vi "ShiftWristSetpoints.vi"(1 "Grab Hatch":bool, 2 "Setpoints":dbl[](array[numeric])) -> (0 "Setpoints Out":dbl[](array[numeric]))   [LabVIEW 2018]
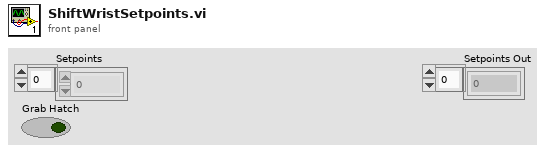
[diagram p1: front panel]
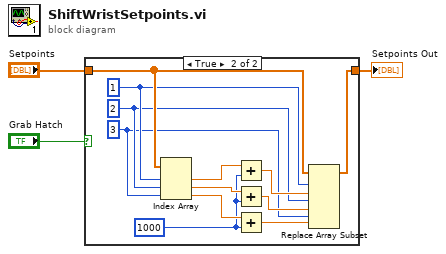
[diagram p0: block diagram]
diagram:
  n1 = case shown="True" "Grab Hatch" {
    tunnel: "Setpoints" -> [w4 w16]
    tunnel: [w4 w5] -> w2
    frame False {
    }
    frame True {
      w12 = 1000
      w6 = 3 ("index")
      w7 = 2 ("index")
      w8 = 1 ("index")
      n2 = Index Array(array=w16, index #1=w8, index #2=w7, index #3=w6) -> (element #1=w15:dbl, element #2=w14:dbl, element #3=w13:dbl)
      n3 = Add(x=w15, y=w12) -> (x+y=w11:dbl)
      n4 = Add(x=w14, y=w12) -> (x+y=w10:dbl)
      n5 = Add(x=w13, y=w12) -> (x+y=w9:dbl)
      n6 = Replace Array Subset(array=w16, new element #1=w11, index #1=w8, new element #2=w10, index #2=w7, new element #3=w9, index #3=w6) -> (w5:dbl[])
    }
  }
  "Setpoints Out" <- w2
